vi "FPGA Image Processing (FPGA).vi"() -> ()   [LabVIEW 2013, in "FPGA Image Processing.lvlib"]
uses:
  FPGA Image Processing.lvlib
  <vilib>/eio/EIONode/EIONode.xnode
  <vilib>/rvi/eio/common/nirviEmuTemplateMethod_errors.vi
  <vilib>/Platform/TimedLoop/XDataNode/wakeup.ctl
  <vilib>/Platform/TimedLoop/XDataNode/XDNodeRunTimeDep.lvlib
  <vilib>/Platform/TimedLoop/XDataNode/nitl_modes.ctl
  <vilib>/Platform/TimedLoop/XDataNode/timing_clust.ctl
  <vilib>/Platform/TimedLoop/XDataNode/XDataNode.xnode
  LabVIEW/Vision/Vision-RIO/Vision-RIO/Common/CL Data to Pixels/10 Tap 8-Bit.vi
  LabVIEW/Vision/Vision-RIO/Vision-RIO/Common/CL Configuration.ctl
  LabVIEW/Vision/Vision-RIO/Vision-RIO/Common/CL Signal Mapping.ctl
panel:
  out "Right Wing Sector Pixel Count":u16[](array[numeric])
  out "Left Wing Sector Pixel Count":u16[](array[numeric])
  in  "Pixel":T1
  in  "Wing ROIs":T2
  out "Right Wing Sector Pixel Values":u8[][](array[numeric])
  out "Left Wing Sector Pixel Values":u8[][](array[numeric])
  in  "NumWingSectors":u8
  in  "UART.Transmit":bool
  in  "UART.Tx Data":u8[](array[numeric])=[0, 0, 0, 0, 0, 0, 0, 0, 0, 0] format="%02x"
  in  "UART.Set Baud Rate":bool
  in  "UART.Byte Mode":bool=TRUE
  out "UART.Rx Ready":bool
  out "UART.Break Indicator":bool
  out "UART.Framing Error":bool
  out "UART.Overrun Error":bool
  out "UART.Tx Ready":bool
  out "UART.Rx Data":u8 format="%02x"
  in  "UART.Receive":bool
  in  "UART.Baud Rate":u8
  in  "Acq Control.Ignore DVAL":bool
  in  "Acq Control.Cancel Acq":bool
  in  "Acq Control.Acquire":bool
  out "Acq Status.Frames Acq'd":u32
  out "Acq Status.Lines Per Frame":u32
  out "Acq Status.Clocks Per Line":u32
  in  "Acq Control.Frames To Acq":u32
  out "Acq Status.Acq In Progress":bool
  in  "Acq Control.Line Scan Height":u32
  in  "Acq Control.Initialize":bool
  out "Acq Status.Initialized":bool
  in  "CL Config.DVAL Active High":bool=TRUE
  in  "CL Config.FVAL Active High":bool=TRUE
  in  "CL Config.LVAL Active High":bool=TRUE
  in  "CL Config.Spare Active High":bool=TRUE
  in  "CL Config.Line Scan":bool
  in  "CL Config.Signal Mapping":T3=enum."Basler 10-tap"
  in  "CL Config.Configuration":T4=enum."Full"
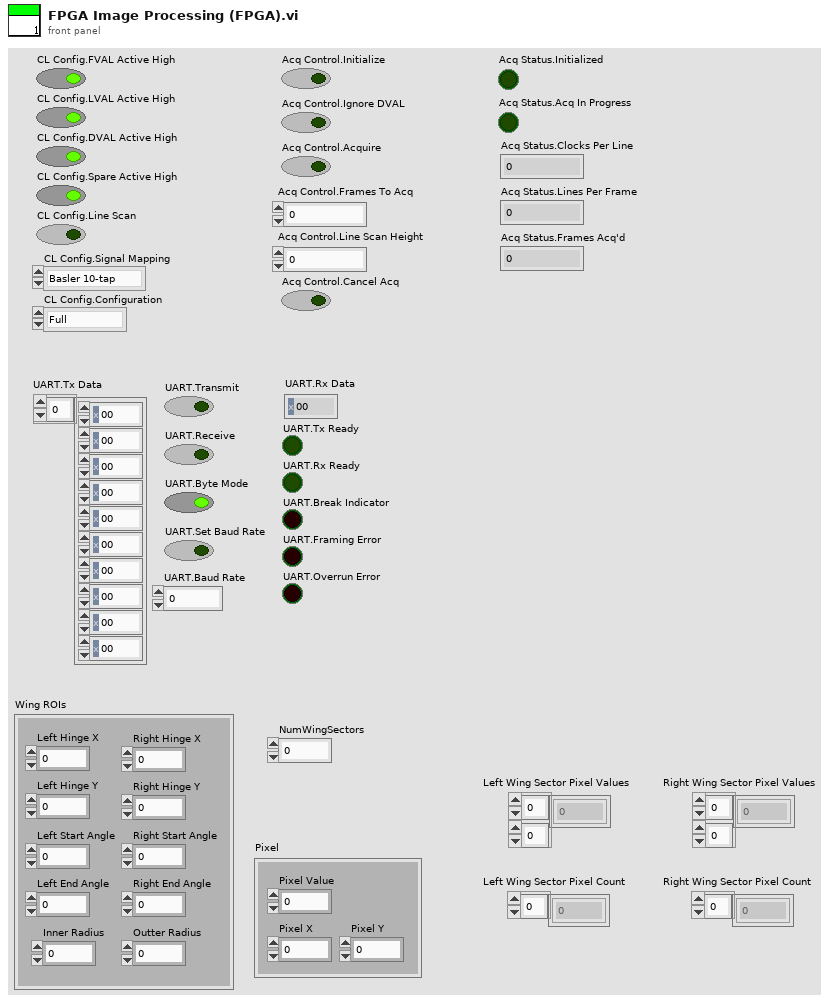
[diagram p1: front panel]
types:
  T1 = cluster{"Pixel Value":u8, "Pixel X":u16, "Pixel Y":u16}
  T2 = cluster{"Left Hinge X":u16, "Left Hinge Y":u16, "Inner Radius":u16, "Outter Radius":u16, "Right Hinge X":u16, "Right Hinge Y":u16, "Right Start Angle":i16, "Right End Angle":i16, "Left Start Angle":i16, "Left End Angle":i16}
  T3 = typedef "CL Signal Mapping.ctl" = enum8{"Standard", "Basler 10-tap", "Vosskühler 10-tap"}
  T4 = typedef "CL Configuration.ctl" = enum8{"Base", "Medium", "Full"}
  T5 = typedef "XDNodeRunTimeDep.lvlib/timing_clust.ctl" = cluster{"Expected End [f-1]":u64, "Actual End [f-1]":u64, "Finished Late? [f-1]":bool, "Expected End [i-1]":u64, "Actual End [i-1]":u64, "Finished Late? [i-1]":bool, "Expected Start [i]":u64, "Actual Start [i]":u64, "Expected Start [f]":u64, "Actual Start [f]":u64, "Source Name":string, "Structure Name":string, "Period":i64, "Deadline":i64, "Offset":i64, "Start":i64, "Priority":i32, "Timeout":i32, "Mode":T6, "Wakeup Reason":T7, "Error":errorcluster, "Source Type":string, "Secondary Source Type":string, "Global End Time":u64, "Global Start Time":u64, "Frame Duration":u64, "Iteration Duration":u64, "Assigned CPU":i32, "I/O Scan Engine Mode":u32}
  T6 = typedef "XDNodeRunTimeDep.lvlib/nitl_modes.ctl" = enum32{"No Change", "Process missed periods, maintain original phase", "Discard missed periods, maintain original phase", "Process missed periods, ignore original phase", "Discard missed periods, ignore original phase"}
  T7 = typedef "XDNodeRunTimeDep.lvlib/wakeup.ctl" = enum32{"Normal", "Aborted", "Asynchronous wakeup", "Timing source error", "Timed loop error", "Timeout"}
  T8 = cluster{"Enables Valid":bool, "Frame Valid":bool, "Line Valid":bool, "Data Valid":bool}
  T9 = cluster{"Pixel 0":u8, "Pixel 1":u8, "Pixel 2":u8, "Pixel 3":u8, "Pixel 4":u8, "Pixel 5":u8, "Pixel 6":u8, "Pixel 7":u8, "Pixel 8":u8, "Pixel 9":u8}
  T10 = cluster{"Tx Data":u8[], "Transmit":bool, "Receive":bool, "Byte Mode":bool, "Set Baud Rate":bool, "Baud Rate":u8}
  T11 = cluster{"Rx Data":u8, "Turn Off Transmit":bool, "Turn Off Receive":bool, "Turn Off Set Baud Rate":bool, "Tx Ready":bool, "Rx Ready":bool, "Break Indicator":bool, "Framing Error":bool, "Overrun Error":bool}
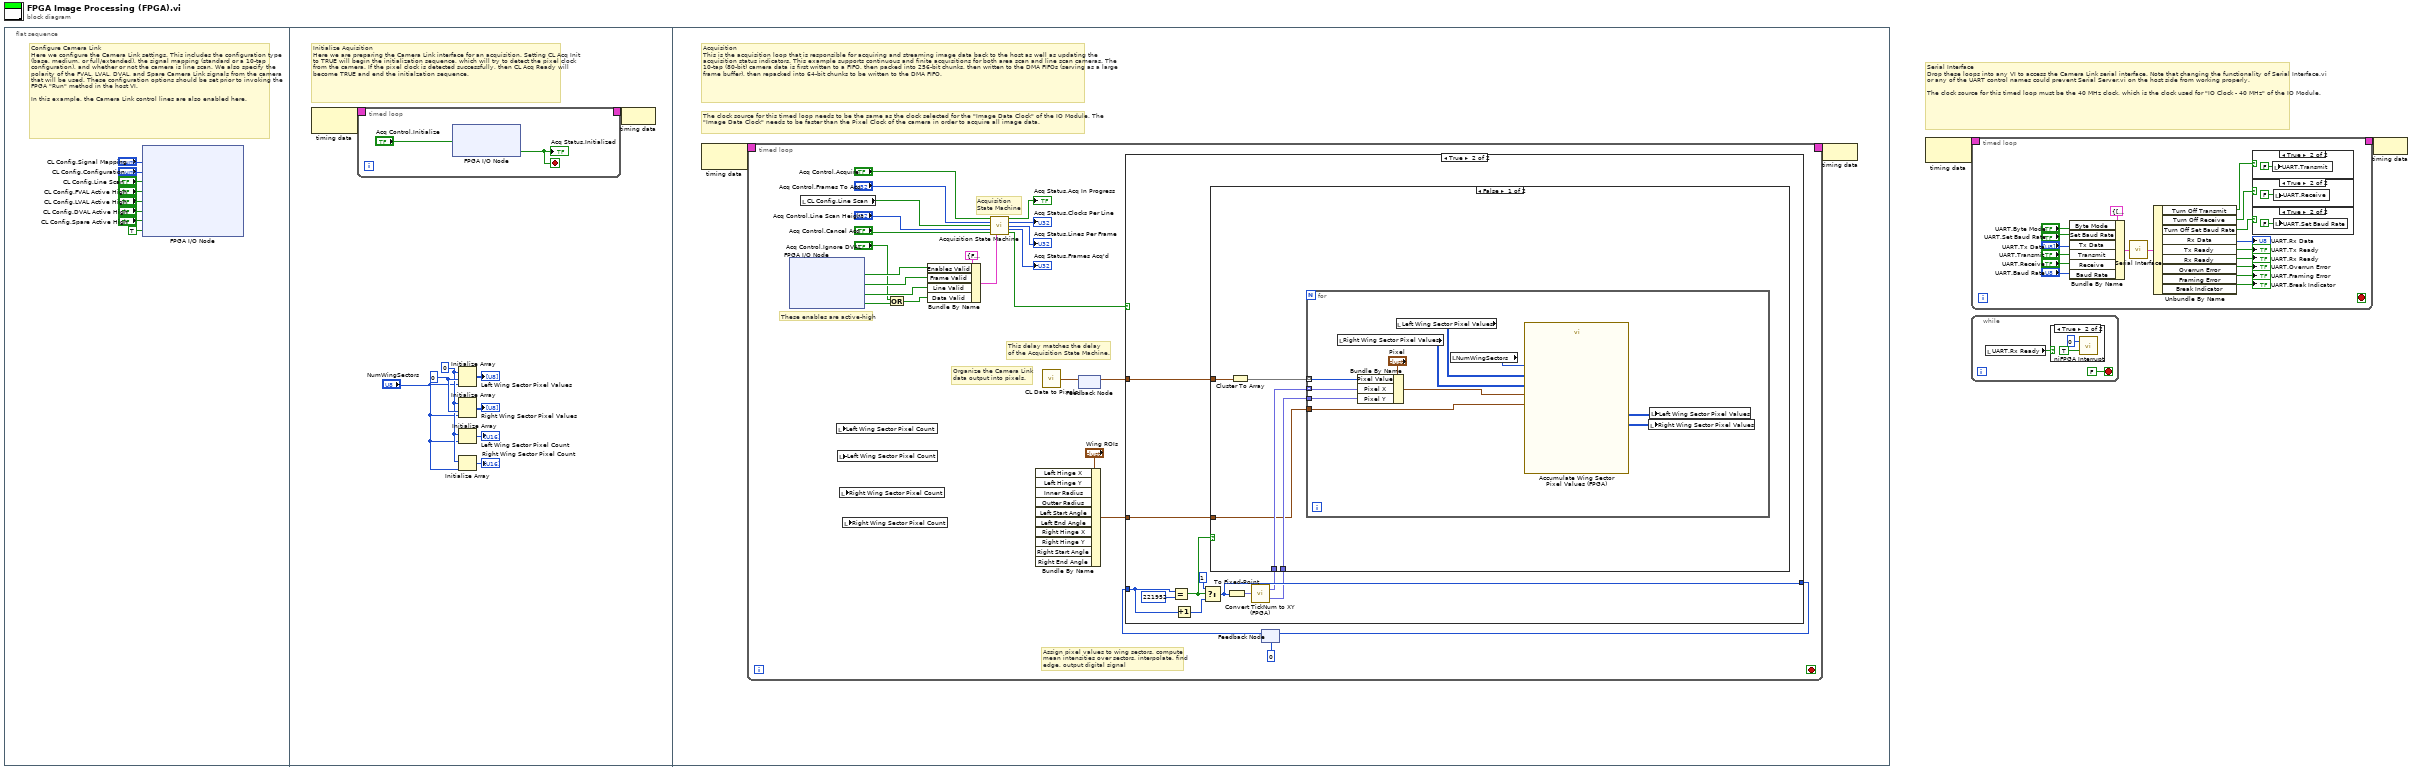
[diagram p0: block diagram]
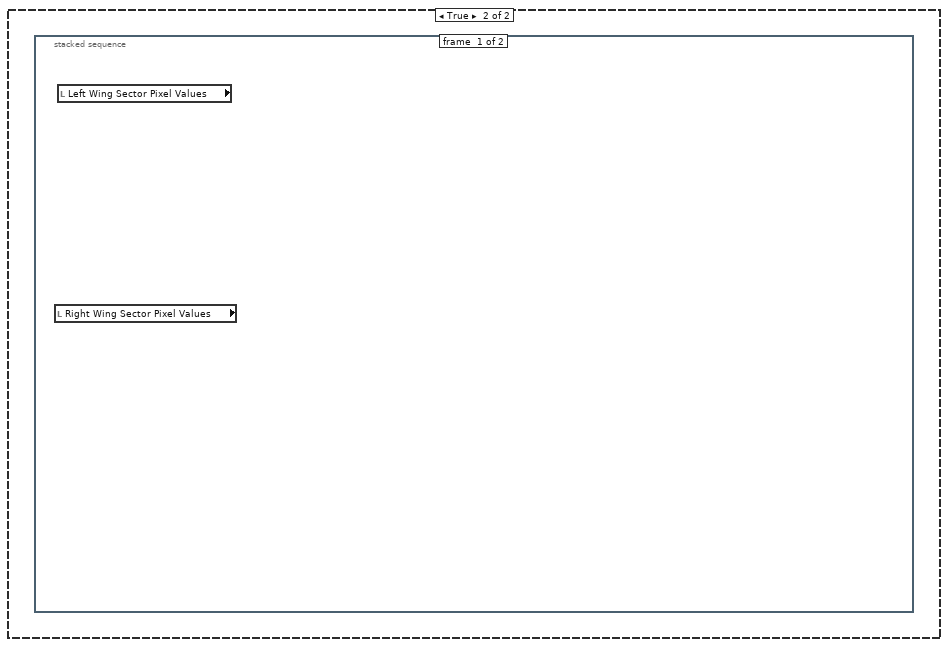
[diagram p7: hidden frame]
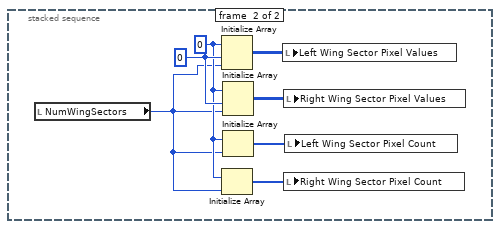
[diagram p8: hidden frame]
diagram:
  # "Serial Interface\nDrop these loops into any VI to access the Camera Link serial interface. Note that changing the functionality of Serial Interface.vi or any of the UART control names could prevent Serial Server.vi on the host side from working properly.\n\nThe clock source for this timed loop must be the 40 MHz clock, which is the clock used for \"IO Clock - 40 MHz\" of the IO Module."
  n1 = flat-sequence {
    frame #0 {
      # "Configure Camera Link\nHere we configure the Camera Link settings. This includes the configuration type (base, medium, or full/extended), the signal mapping (standard or a 10-tap configuration), and whether or not the camera is line scan. We also specify the polarity of the FVAL, LVAL, DVAL, and Spare Camera Link signals from the camera that will be used. These configuration options should be set prior to invoking the FPGA \"Run\" method in the host VI.\n\nIn this example, the Camera Link control lines are also enabled here."
      n2 = xnode "FPGA I/O Node"("CL Set Signal Mapping"="CL Config.Signal Mapping", "CL Set Configuration"="CL Config.Configuration", "CL Set Line Scan"="CL Config.Line Scan", "CL Set FVAL Active High"="CL Config.FVAL Active High", "CL Set LVAL Active High"="CL Config.LVAL Active High", "CL Set DVAL Active High"="CL Config.DVAL Active High", "CL Set Spare Active High"="CL Config.Spare Active High", "CL Control Enable"=TRUE ("IO Module\\CL Control Enable")) -> ()  [unwired: 8 in, 8 out]
    }
    frame #1 {
      w16 = 0 ("dimension size")
      w12 = u8 0 ("element")
      # "Initialize Aquisition\nHere we are preparing the Camera Link interface for an acquisition. Setting CL Acq Init to TRUE will begin the initialization sequence, which will try to detect the pixel clock from the camera. If the pixel clock is detected successfully, then CL Acq Ready will become TRUE and end the initialzation sequence."
      n3 = node-c288() -> (w19:T5)  [unwired: 1 out]
      n4 = timed-loop {
        timing: w19 -> [_]
        timing-out: [_] -> w18
        stop <- w20 stop-if-true
        n5 = xnode "FPGA I/O Node"("CL Acq Init"="Acq Control.Initialize") -> ("CL Acq Ready"=w20:bool)  [unwired: 2 in, 2 out]
        "Acq Status.Initialized" <- w20
      }
      n6 = Initialize Array(w12, w16, "NumWingSectors") -> (→"Left Wing Sector Pixel Values":u8[][])
      n7 = Initialize Array(w12, w16, "NumWingSectors") -> (→"Right Wing Sector Pixel Values":u8[][])
      n8 = Initialize Array(w12, "NumWingSectors") -> (→"Left Wing Sector Pixel Count":u8[])
      n9 = Initialize Array(w12, "NumWingSectors") -> (→"Right Wing Sector Pixel Count":u8[])
      n10 = node-c288(w18) -> ()
    }
    frame #2 {
      # "The clock source for this timed loop needs to be the same as the clock selected for the \"Image Data Clock\" of the IO Module. The \"Image Data Clock\" needs to be faster than the Pixel Clock of the camera in order to acquire all image data."
      # "Acquisition\nThis is the acquisition loop that is responsible for acquiring and streaming image data back to the host as well as updating the acquisition status indicators. This example supports continuous and finite acquisitions for both area scan and line scan cameras. The 10-tap (80-bit) camera data is first written to a FIFO, then packed into 256-bit chunks, then written to the DMA FIFOs (serving as a large frame buffer), then repacked into 64-bit chunks to be written to the DMA FIFO."
      n11 = node-c288() -> (w27:T5)  [unwired: 1 in]
      n12 = timed-loop {
        timing: w27 -> [_]
        timing-out: [_] -> w26
        stop <- _ stop-if-true
        # "Assign pixel values to wing sectors, compute\nmean intensities over sectors, interpolate, find\nedge, output digital signal"
        # "Organize the Camera Link\ndata output into pixels."
        # "These enables are active-high"
        # "This delay matches the delay\nof the Acquisition State Machine."
        # "Acquisition\nState Machine"
        n13 = xnode "FPGA I/O Node"() -> ("CL Output Valid"=w44:bool, "CL Frame Valid"=w43:bool, "CL Line Valid"=w42:bool, "CL Data Valid"=w39:bool)  [unwired: 4 in, 4 out]
        n14 = local read "CL Config.Line Scan"() -> (w36:bool)
        n15 = local read "Left Wing Sector Pixel Count"() -> ()  [unwired: 1 in]
        n16 = local read "Left Wing Sector Pixel Count"() -> ()  [unwired: 1 in]
        n17 = local read "Right Wing Sector Pixel Count"() -> ()  [unwired: 1 in]
        n18 = local read "Right Wing Sector Pixel Count"() -> ()  [unwired: 1 in]
        n19 = Or(x="Acq Control.Ignore DVAL", y=w39) -> (x .or. y?=w38:bool)
        n20 = Bundle By Name(cluster=T8 {"Enables Valid"=FALSE, "Frame Valid"=FALSE, "Line Valid"=FALSE, "Data Valid"=FALSE} ("Enables"), "Enables Valid"=w44, "Frame Valid"=w43, "Line Valid"=w42, "Data Valid"=w38) -> (w41:T8)
        n21 = call "Acquisition State Machine.vi"("Acquire"="Acq Control.Acquire", "Frames to Acquire"="Acq Control.Frames To Acq", "Line Scan"=w36, "Line Scan Height"="Acq Control.Line Scan Height", "Cancel Acq"="Acq Control.Cancel Acq", "Enables"=w41) -> ("Acq In Progress"=→"Acq Status.Acq In Progress":bool, "Num Clocks Per Line"=→"Acq Status.Clocks Per Line":u32, "Num Lines Per Frame"=→"Acq Status.Lines Per Frame":u32, "Num Frames Acq'd"=→"Acq Status.Frames Acq'd":u32, "Capture Cycle"=w52:bool)  [unwired: 4 in, 1 out]
        n22 = Bundle By Name(cluster="Wing ROIs") -> (w28:T2)  [unwired: 10 in]
        n23 = call-poly "CL Data to Pixels.vi"() -> ("Pixels"=w31:T9)  [unwired: 1 in]
        n24 = feedback #1() -> (w30:T9)  [unwired: 1 in]
        n25 = feedback-in #1(w31) -> ()
        n26 = feedback #2(u32 0 ("y")) -> (w33:u32)
        n27 = case shown="True" w52 {
          tunnel: w33 -> [w53 w63]
          tunnel: [w53 w60] -> w34
          tunnel: w30 -> [_ w56]
          tunnel: w28 -> [_ w54]
          frame False {
          }
          frame True {
            n28 = Equal?(x=w63, y=u32 221952) -> (x = y?=w58:bool)
            n29 = Increment(x=w63) -> (x+1=w61:u32)
            n30 = Select(t=u32 1 ("y"), s=w58, f=w61) -> (s? t:f=w60:u32)
            n31 = To Fixed-Point(number=w60) -> (fixed-point=w59:fxp<+,32,32>)  [unwired: 1 in]
            n32 = call "Convert TickNum to XY (FPGA).vi"("numAcqTick"=w59) -> ("PixelXArray"=w57:fxp<+,1,1>[], "PixelY"=w55:fxp<+,12,12>)
            n33 = case shown="False" w58 {
              tunnel: w57 -> [w68 _]
              tunnel: w56 -> [w69 _]
              tunnel: w55 -> [w67 _]
              tunnel: w54 -> [w65 _]
              frame False {
                n34 = Cluster To Array(cluster=w69) -> (array=w66:u8[])
                n35 = for {
                  tunnel: w68 -> [w78] mode=indexing
                  tunnel: w67 -> [w77]
                  tunnel: w66 -> [w76] mode=indexing
                  tunnel: w65 -> [w75]
                  n36 = local read "Right Wing Sector Pixel Values"() -> (w71:u8[][])
                  n37 = Bundle By Name(cluster="Pixel", "Pixel Value"=w76, "Pixel X"=w78, "Pixel Y"=w77) -> (w79:T1)
                  n38 = local read "Left Wing Sector Pixel Values"() -> (w73:u8[][])
                  n39 = local read "NumWingSectors"() -> (w74:u8)
                  n40 = call "Accumulate Wing Sector Pixel Values (FPGA).vi"("NumWingSectors"=w74, "Right Wing Sector Pixels"=w71, "Left Wing Sector Pixels"=w73, "Wing ROIs"=w75, "Pixel"=w79) -> ("Right Wing Sector Pixels 2"=w70:u8[][], "Left Wing Sector Pixels 2"=w72:u8[][])  [unwired: 2 in, 2 out]
                  n41 = local write "Right Wing Sector Pixel Values"(w70) -> ()
                  n42 = local write "Left Wing Sector Pixel Values"(w72) -> ()
                }
              }
              frame True {
                n43 = stacked-sequence {
                  frame #0 {
                    n44 = local read "Right Wing Sector Pixel Values"() -> ()  [unwired: 1 out]
                    n45 = local read "Left Wing Sector Pixel Values"() -> ()  [unwired: 1 out]
                  }
                  frame #1 {
                    w87 = 0 ("dimension size")
                    w86 = u8 0 ("element")
                    n46 = local read "NumWingSectors"() -> (w85:u8)
                    n47 = Initialize Array(w86, w87, w85) -> (w84:u8[][])
                    n48 = Initialize Array(w86, w85) -> (w81:u8[])
                    n49 = Initialize Array(w86, w87, w85) -> (w83:u8[][])
                    n50 = Initialize Array(w86, w85) -> (w82:u8[])
                    n51 = local write "Left Wing Sector Pixel Values"(w84) -> ()
                    n52 = local write "Right Wing Sector Pixel Values"(w83) -> ()
                    n53 = local write "Right Wing Sector Pixel Count"(w81) -> ()
                    n54 = local write "Left Wing Sector Pixel Count"(w82) -> ()
                  }
                }
              }
            }
          }
        }
        n55 = feedback-in #2(w34) -> ()
      }
      n56 = node-c288(w26) -> ()
    }
  }
  n57 = node-c288() -> (w2:T5)  [unwired: 1 out]
  n58 = timed-loop {
    timing: w2 -> [_]
    timing-out: [_] -> w1
    stop <- _ stop-if-true
    n59 = Bundle By Name(cluster=T10 {"Tx Data"=[0, 0, 0, 0, 0, 0, 0, 0, 0, 0], "Transmit"=FALSE, "Receive"=FALSE, "Byte Mode"=TRUE, "Set Baud Rate"=FALSE, "Baud Rate"=0} ("UART Inputs"), "Byte Mode"="UART.Byte Mode", "Set Baud Rate"="UART.Set Baud Rate", "Tx Data"="UART.Tx Data", "Transmit"="UART.Transmit", "Receive"="UART.Receive", "Baud Rate"="UART.Baud Rate") -> (w92:T10)
    n60 = call "Serial Interface.vi"("UART Inputs"=w92) -> ("UART Outputs"=w104:T11)
    n61 = Unbundle By Name(w104) -> ("Turn Off Transmit"=w97:bool, "Turn Off Receive"=w98:bool, "Turn Off Set Baud Rate"=w94:bool, "Rx Data"=→"UART.Rx Data":u8, "Tx Ready"=→"UART.Tx Ready":bool, "Rx Ready"=→"UART.Rx Ready":bool, "Overrun Error"=→"UART.Overrun Error":bool, "Framing Error"=→"UART.Framing Error":bool, "Break Indicator"=→"UART.Break Indicator":bool)
    n62 = case shown="True" w97 {
      frame False {
      }
      frame True {
        n63 = local write "UART.Transmit"(FALSE ("UART.Transmit")) -> ()
      }
    }
    n64 = case shown="True" w98 {
      frame False {
      }
      frame True {
        n65 = local write "UART.Receive"(FALSE ("UART.Receive")) -> ()
      }
    }
    n66 = case shown="True" w94 {
      frame False {
      }
      frame True {
        n67 = local write "UART.Set Baud Rate"(FALSE ("UART.Receive")) -> ()
      }
    }
  }
  n68 = while {
    stop <- FALSE stop-if-true
    n69 = local read "UART.Rx Ready"() -> (w116:bool)
    n70 = case shown="True" w116 {
      frame False {
      }
      frame True {
        n71 = call <vilib>:"niFPGA Interrupt.vi"("Wait Until Cleared (F)"=TRUE ("Wait Until Cleared"), "IRQ Number (0)"=u8 0 ("IRQ Number")) -> ()  [unwired: 1 in]
      }
    }
  }
  n72 = node-c288(w1) -> ()
